vi "Receive TCP Message HMI devices.vi"(4 "error in (no error)":errorcluster, 5 "TCP Joystick Ref In":refnum<k5>, 7 "Supervisor in":refnum<class "Supervisor.lvclass">) -> (0 "error out":errorcluster, 1 "TCP Joystick Ref Out":refnum<k5>, 2 "Exit":bool, 3 "Supervisor out":refnum<class "Supervisor.lvclass">)   [LabVIEW 2014, in "Supervisor.lvclass"]
uses:
  Supervisor.lvclass
panel:
  out "data out":string
  out "error out 4":errorcluster
  out "error out 3":errorcluster
  out "error out 2":errorcluster
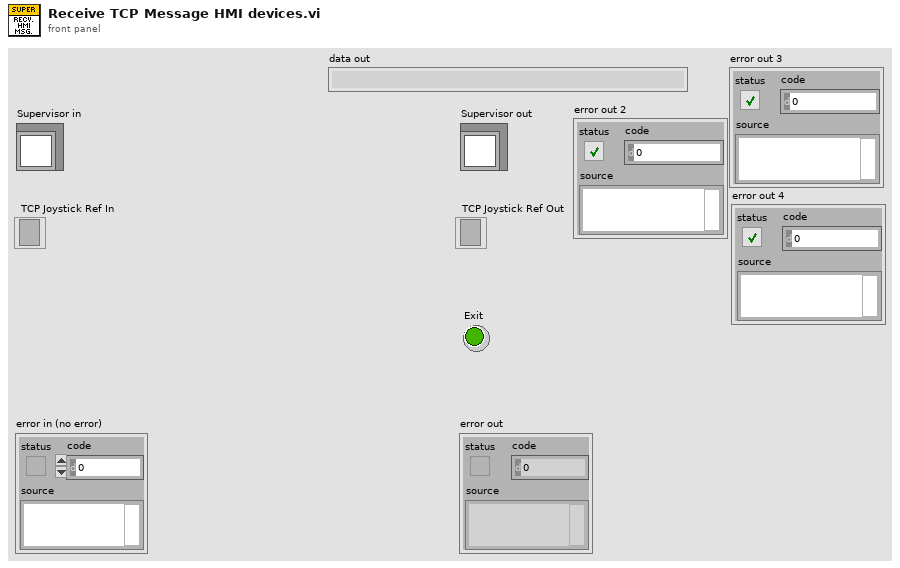
[diagram p1: front panel]
types:
  T1 = cluster{"Axis Translation":cluster{"X-Axis":dbl, "Y-Axis":dbl, "Z-Axis":dbl}, "Axis Rotation":cluster{"X-Axis":dbl, "Y-Axis":dbl, "Z-Axis":dbl}}
  T2 = cluster{"Button 1":bool, "Button 2":bool, "Button 3":bool, "Button 4":bool, "Button 5":bool, "Button 6":bool, "Button 7":bool, "Button 8":bool, "Button 9":bool, "Button 10":bool, "Button 11":bool, "Button 12":bool, "POV Direction":i32}
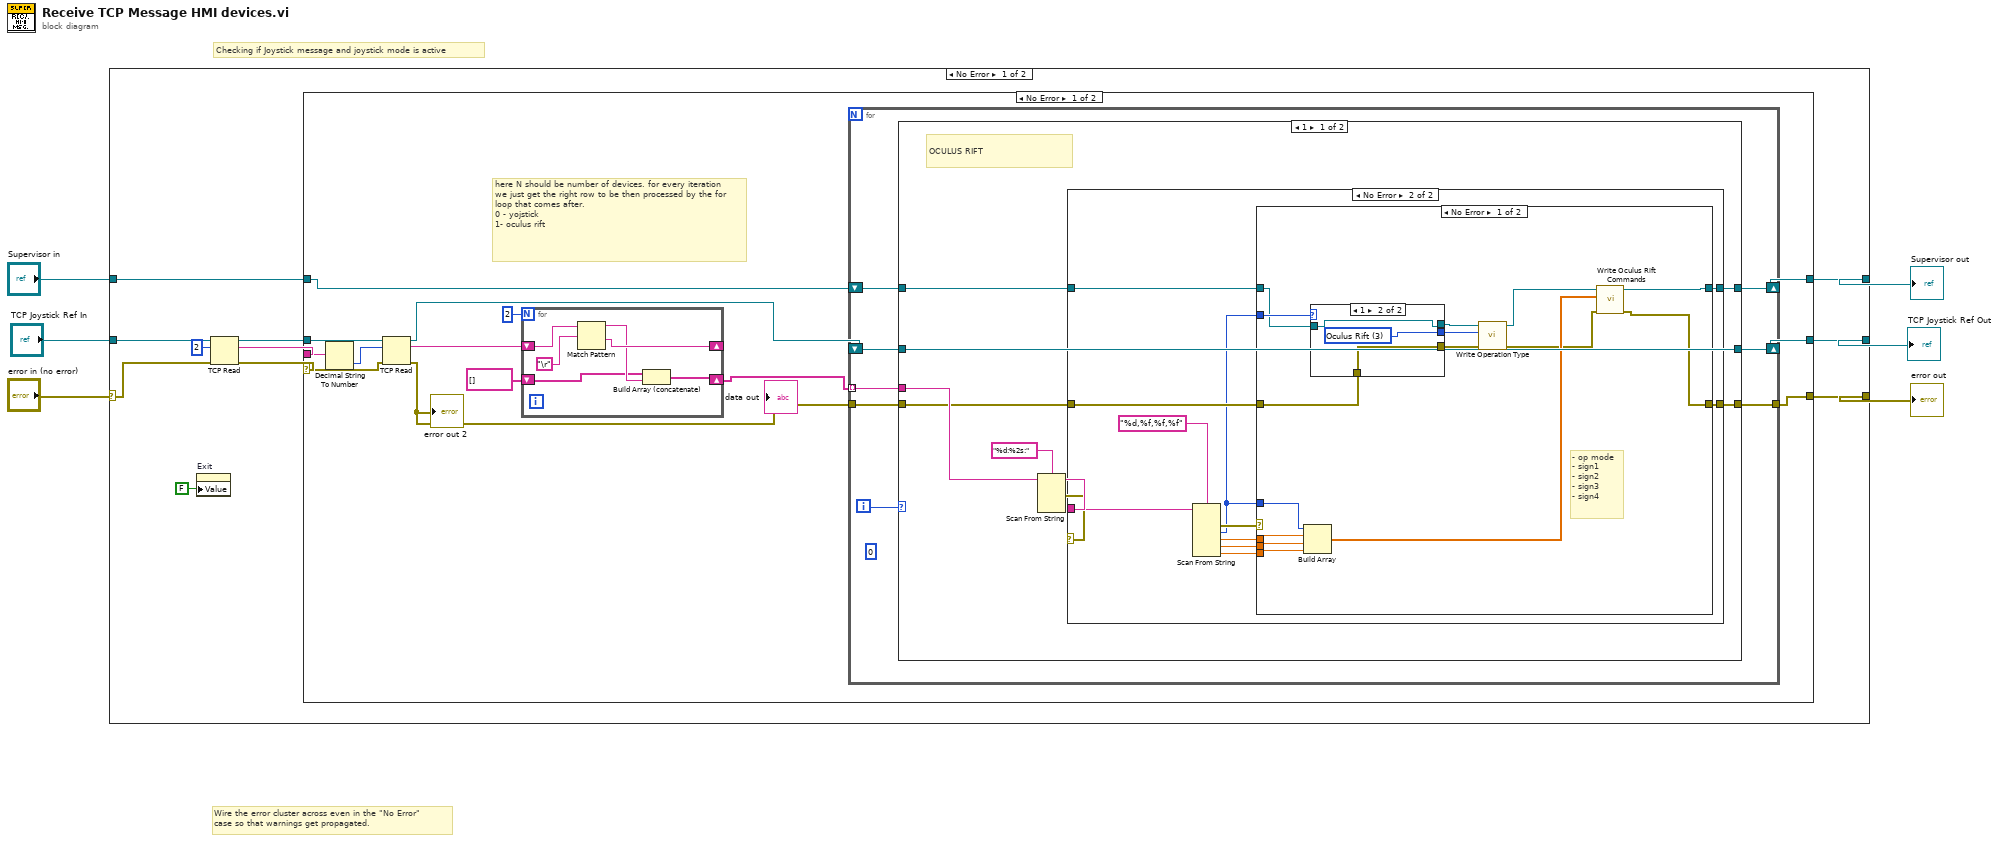
[diagram p0: block diagram]
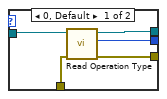
[diagram p3: hidden frame]
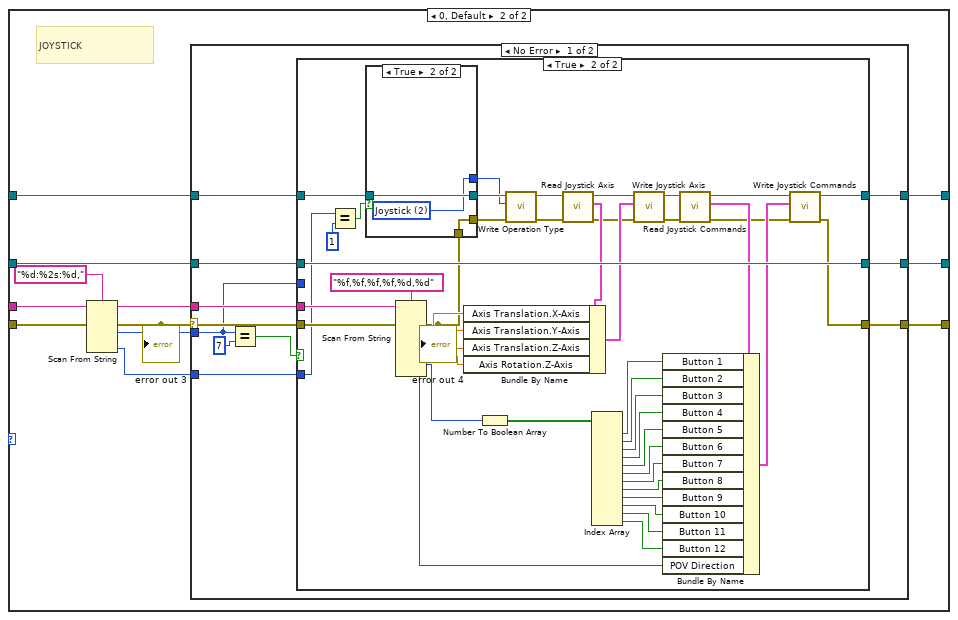
[diagram p5: hidden frame]
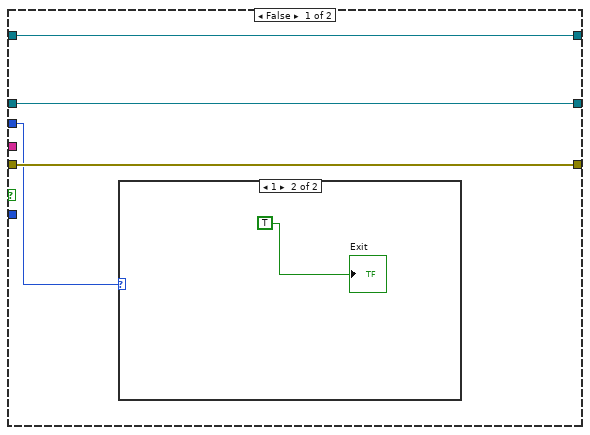
[diagram p6: hidden frame]
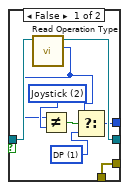
[diagram p8: hidden frame]
diagram:
  # "Checking if Joystick message and joystick mode is active"
  # "Wire the error cluster across even in the \"No Error\"\ncase so that warnings get propagated."
  n1 = case shown="No Error" "error in (no error)" {
    selector: "error in (no error)" -> [w13 w185]
    tunnel: [w11 w185] -> w5
    tunnel: [w14 w184] -> w3
    tunnel: "Supervisor in" -> [w15 w184]
    tunnel: "TCP Joystick Ref In" -> [w17 w183]
    tunnel: [w12 w183] -> w1
    frame No Error {
      n2 = property on="Exit" class="Bool (strict)"("Value"=FALSE ("Exit")) -> ()  [unwired: 2 in, 2 out]
      n3 = TCP Read(connection ID=w17, bytes to read=2, error in (no error)=w13) -> (connection ID out=w16:refnum<k5>, data out=w8:string, error out=w10:errorcluster)  [unwired: 2 in]
      n4 = case shown="No Error" w10 {
        selector: w10 -> [w26 w180]
        tunnel: w8 -> [w23 _]
        tunnel: w16 -> [w31 w181]
        tunnel: w15 -> [w30 w182]
        tunnel: [w29 w182] -> w14
        tunnel: [w27 w181] -> w12
        tunnel: [w24 w180] -> w11
        frame No Error {
          # "here N should be number of devices. for every iteration we just get the right row to be then processed by the for loop that comes after.\n0 - yojstick\n1- oculus rift"
          n5 = Decimal String To Number(string=w23) -> (number=w21:i32)  [unwired: 2 in, 1 out]
          n6 = TCP Read(connection ID=w31, bytes to read=w21, error in (no error)=w26) -> (connection ID out=w28:refnum<k5>, data out=w22:string, error out=w25:errorcluster)  [unwired: 2 in]
          "error out 2" <- w25
          n7 = for {
            N: 2 -> [_]
            shift-right: [w37] -> _
            shift-left: w22 -> [w36]
            shift-right: [w33] -> w18
            shift-left: string[] [] -> [w32]
            n8 = Match Pattern(string=w36, regular expression="\r") -> (before substring=w34:string, after substring=w37:string)  [unwired: 1 in, 2 out]
            n9 = Build Array (concatenate)(w32, w34) -> (w33:string[])
          }
          n10 = for {
            tunnel: w18 -> [w41] mode=indexing
            shift-right: [w44] -> w29
            shift-left: w30 -> [w45]
            shift-right: [w42] -> w27
            shift-left: w28 -> [w43]
            tunnel: [w40] -> w24
            tunnel: w25 -> [w39]
            i -> [w38]
            (unwired) 0
            n11 = case shown="1" w38 {
              tunnel: w45 -> [w50 w101]
              tunnel: [w49 w100] -> w44
              tunnel: w39 -> [w48 w99]
              tunnel: w43 -> [w54 w97]
              tunnel: [w54 w96] -> w42
              tunnel: [w47 w95] -> w40
              tunnel: w41 -> [w52 w94]
              frame 1 {
                # "OCULUS RIFT"
                n12 = Scan From String(format string="%d:%2s:", input string=w52) -> (remaining string=w51:string, error out=w46:errorcluster)  [unwired: 6 in, 1 out]
                n13 = case shown="No Error" w46 {
                  tunnel: w51 -> [_ w67]
                  tunnel: w50 -> [w55 w62]
                  tunnel: [w55 w61] -> w49
                  tunnel: w48 -> [w56 w60]
                  tunnel: [w56 w59] -> w47
                  frame Error {
                  }
                  frame No Error {
                    n14 = Scan From String(format string="%d,%f,%f,%f", input string=w67) -> (error out=w58:errorcluster, output 1=w57:i32, output 2=w65:dbl, output 3=w64:dbl, output 4=w63:dbl)  [unwired: 6 in, 2 out]
                    n15 = case shown="No Error" w58 {
                      tunnel: w65 -> [w82 _]
                      tunnel: w64 -> [w81 _]
                      tunnel: w63 -> [w80 _]
                      tunnel: w62 -> [w73 w92]
                      tunnel: [w70 w92] -> w61
                      tunnel: w60 -> [w77 w91]
                      tunnel: [w69 w91] -> w59
                      tunnel: w57 -> [w78 _]
                      tunnel: w57 -> [w71 _]
                      frame No Error {
                        # "- op mode\n- sign1\n- sign2\n- sign3\n- sign4"
                        n16 = Build Array(w71, w82, w81, w80) -> (w79:dbl[])
                        n17 = case shown="1" w78 {
                          tunnel: [w87 w88] -> w68
                          tunnel: w77 -> [w86 w89]
                          tunnel: [w85 w89] -> w76
                          tunnel: [w84 w90] -> w74
                          tunnel: w73 -> [w83 w90]
                          frame 0, Default {
                            n18 = call-dynamic "Read Operation Type.vi"("error in (no error)"=w86, "Supervisor in"=w83) -> ("error out"=w85:errorcluster, "Operation Type"=w87:u16, "Supervisor out"=w84:refnum<class "Supervisor.lvclass">)  [unwired: 7 in]
                          }
                          frame 1 {
                            w88 = u16 3 items=["Tracking", "DP", "Joystick", "Oculus Rift"] ("Operation Type")
                          }
                        }
                        n19 = call-dynamic "Write Operation Type.vi"("error in (no error)"=w76, "Operation Type"=w68, "Supervisor in"=w74) -> ("error out"=w75:errorcluster, "Supervisor out"=w72:refnum<class "Supervisor.lvclass">)  [unwired: 7 in]
                        n20 = call-dynamic "Write Oculus Rift Commands.vi"("error in (no error)"=w75, "Oculus Rift Commands"=w79, "Supervisor in"=w72) -> ("error out"=w69:errorcluster, "Supervisor out"=w70:refnum<class "Supervisor.lvclass">)  [unwired: 7 in]
                      }
                      frame Error {
                      }
                    }
                  }
                }
              }
              frame 0, Default {
                # "JOYSTICK"
                n21 = Scan From String(format string="%d:%2s:%d,", input string=w94, error in=w99) -> (remaining string=w103:string, error out=w98:errorcluster, output 1=w102:i32, output 3=w93:i32)  [unwired: 5 in, 1 out]
                "error out 3" <- w98
                n22 = case shown="No Error" w98 {
                  selector: w98 -> [w109 w177]
                  tunnel: w103 -> [w115 _]
                  tunnel: w93 -> [w107 _]
                  tunnel: w102 -> [w105 _]
                  tunnel: w101 -> [w113 w179]
                  tunnel: [w112 w179] -> w100
                  tunnel: w97 -> [w111 w178]
                  tunnel: [w110 w178] -> w96
                  tunnel: [w108 w177] -> w95
                  frame No Error {
                    n23 = Equal?(x=w105, y=7) -> (x = y?=w106:bool)
                    n24 = case shown="True" w106 {
                      tunnel: w115 -> [_ w164]
                      tunnel: w113 -> [w116 w130]
                      tunnel: [w116 w133] -> w112
                      tunnel: w111 -> [w119 w165]
                      tunnel: [w119 w165] -> w110
                      tunnel: w109 -> [w118 w155]
                      tunnel: [w118 w132] -> w108
                      tunnel: w107 -> [_ w127]
                      tunnel: w105 -> [w117 _]
                      frame False {
                        n25 = case shown="1" w117 {
                          frame 0, Default {
                          }
                          frame 1 {
                            "Exit" <- TRUE ("Exit Flag")
                          }
                        }
                      }
                      frame True {
                        n26 = Equal?(x=w127, y=1) -> (x = y?=w122:bool)
                        n27 = Scan From String(format string="%f,%f,%f,%f,%d,%d", input string=w164, error in=w155) -> (error out=w129:errorcluster, output 1=w161:dbl, output 2=w160:dbl, output 3=w159:dbl, output 4=w158:dbl, output 5=w153:i32, output 6=w149:i32)  [unwired: 7 in, 2 out]
                        "error out 4" <- w129
                        n28 = case shown="True" w122 {
                          tunnel: w130 -> [w172 w176]
                          tunnel: [w171 w176] -> w126
                          tunnel: w129 -> [w173 w175]
                          tunnel: [w173 w175] -> w123
                          tunnel: [w166 w174] -> w121
                          frame False {
                            w168 = u16 1 items=["Tracking", "DP", "Joystick", "Oculus Rift"] ("Operation Type")
                            w169 = u16 2 items=["Tracking", "DP", "Joystick", "Oculus Rift"] ("Operation Type")
                            n29 = call-dynamic "Read Operation Type.vi"("Supervisor in"=w172) -> ("Operation Type"=w167:u16, "Supervisor out"=w171:refnum<class "Supervisor.lvclass">)  [unwired: 8 in, 1 out]
                            n30 = Not Equal?(x=w167, y=w169) -> (x != y?=w170:bool)
                            n31 = Select(t=w167, s=w170, f=w168) -> (s? t:f=w166:u16)
                          }
                          frame True {
                            w174 = u16 2 items=["Tracking", "DP", "Joystick"] ("Operation Type")
                          }
                        }
                        n32 = Number To Boolean Array(number=w153) -> (Boolean array=w148:bool[])
                        n33 = call-dynamic "Write Operation Type.vi"("error in (no error)"=w123, "Operation Type"=w121, "Supervisor in"=w126) -> ("error out"=w124:errorcluster, "Supervisor out"=w125:refnum<class "Supervisor.lvclass">)  [unwired: 7 in]
                        n34 = call-dynamic "Read Joystick Axis.vi"("error in (no error)"=w124, "Supervisor in"=w125) -> ("error out"=w154:errorcluster, "Joystick Axis"=w162:T1, "Supervisor out"=w156:refnum<class "Supervisor.lvclass">)  [unwired: 7 in]
                        n35 = Bundle By Name(cluster=w162, "Axis Translation.X-Axis"=w161, "Axis Translation.Y-Axis"=w160, "Axis Translation.Z-Axis"=w159, "Axis Rotation.Z-Axis"=w158) -> (w157:T1)
                        n36 = Index Array(array=w148) -> (element #1=w147:bool, element #2=w146:bool, element #3=w145:bool, element #4=w144:bool, element #5=w143:bool, element #6=w142:bool, element #7=w141:bool, element #8=w140:bool, element #9=w139:bool, element #10=w138:bool, element #11=w137:bool, element #12=w136:bool)  [unwired: 12 in]
                        n37 = call-dynamic "Write Joystick Axis.vi"("error in (no error)"=w154, "Joystick Axis"=w157, "Supervisor in"=w156) -> ("error out"=w151:errorcluster, "Supervisor out"=w152:refnum<class "Supervisor.lvclass">)  [unwired: 7 in]
                        n38 = call-dynamic "Read Joystick Commands.vi"("error in (no error)"=w151, "Supervisor in"=w152) -> ("error out"=w131:errorcluster, "Joystick Commands"=w135:T2, "Supervisor out"=w150:refnum<class "Supervisor.lvclass">)  [unwired: 7 in]
                        n39 = Bundle By Name(cluster=w135, "Button 1"=w147, "Button 2"=w146, "Button 3"=w145, "Button 4"=w144, "Button 5"=w143, "Button 6"=w142, "Button 7"=w141, "Button 8"=w140, "Button 9"=w139, "Button 10"=w138, "Button 11"=w137, "Button 12"=w136, "POV Direction"=w149) -> (w134:T2)
                        n40 = call-dynamic "Write Joystick Commands.vi"("error in (no error)"=w131, "Joystick Commands"=w134, "Supervisor in"=w150) -> ("error out"=w132:errorcluster, "Supervisor out"=w133:refnum<class "Supervisor.lvclass">)  [unwired: 7 in]
                      }
                    }
                  }
                  frame Error {
                  }
                }
              }
            }
          }
        }
        frame Error {
        }
      }
    }
    frame Error {
    }
  }
  "error out" <- w5
  "Supervisor out" <- w3
  "TCP Joystick Ref Out" <- w1
